vi "第六题a.vi"() -> ()   [LabVIEW 2017]
panel:
  in  "停止 2":bool
  out "显示面板":T1 {"油量" scale=0.0..10.0; "转速（转/秒）" scale=0.0..10000.0; "时速（公里/小时）" scale=0.0..280.0}
  in  "控制面板":T2 {"档位" scale=0.0..10.0; "油门" scale=0.0..100.0}
  out "鞍点":string
  out "随机数数组":dbl[][](array[numeric])
  out "字符串":string
  out "报警灯":bool
  in  "开启报警":bool
  in  "报警上线":dbl(slide) scale=0.0..100.0
  out "温度计":dbl(slide) scale=0.0..100.0
  in  "停止":bool
  # "第二题"
  # "第一题"
  # "第三题"
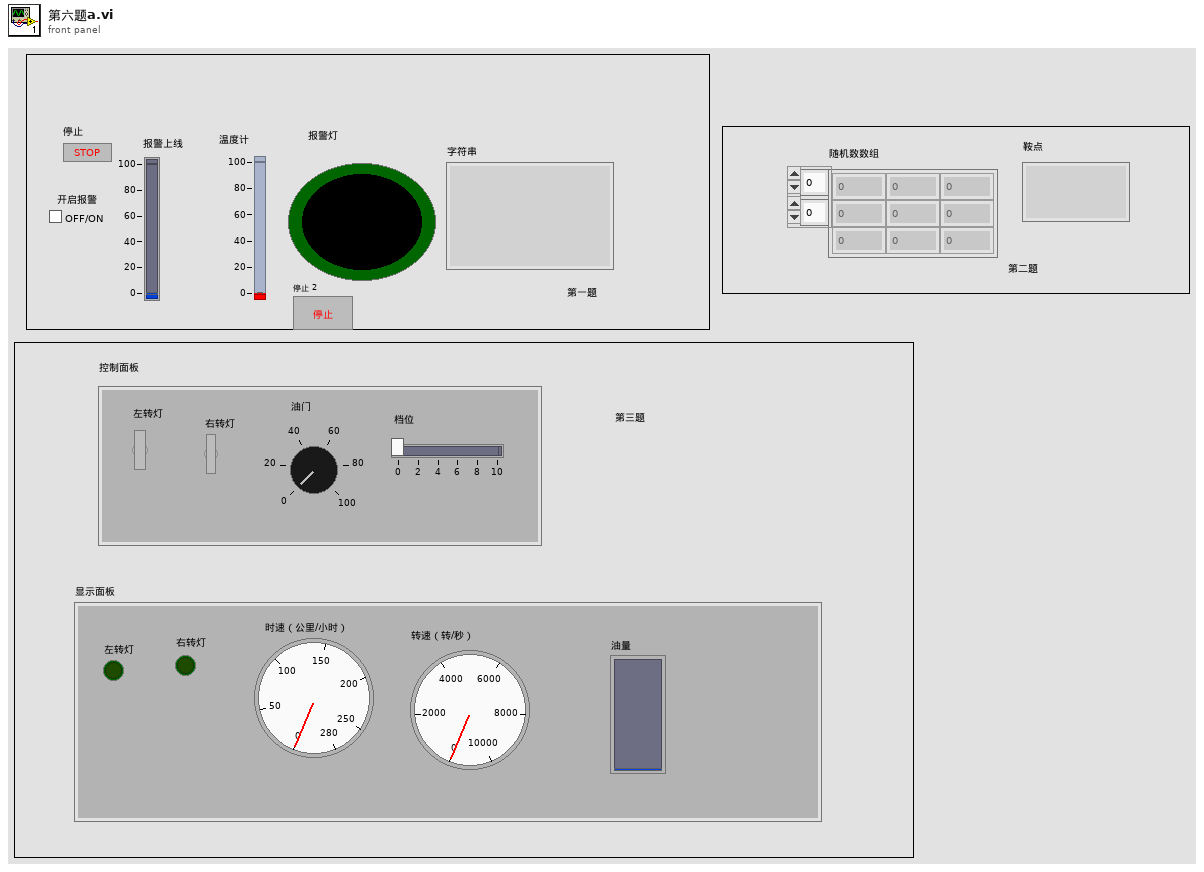
[diagram p1: front panel]
types:
  T1 = cluster{"左转灯":bool, "右转灯":bool, "时速（公里/小时）":dbl, "转速（转/秒） ":dbl, "油量":dbl}
  T2 = cluster{"左转灯":bool, "右转灯":bool, "油门":dbl, "档位":dbl}
  T3 = cluster{"左转灯":bool, "右转灯":bool, dbl, dbl, "b":dbl}
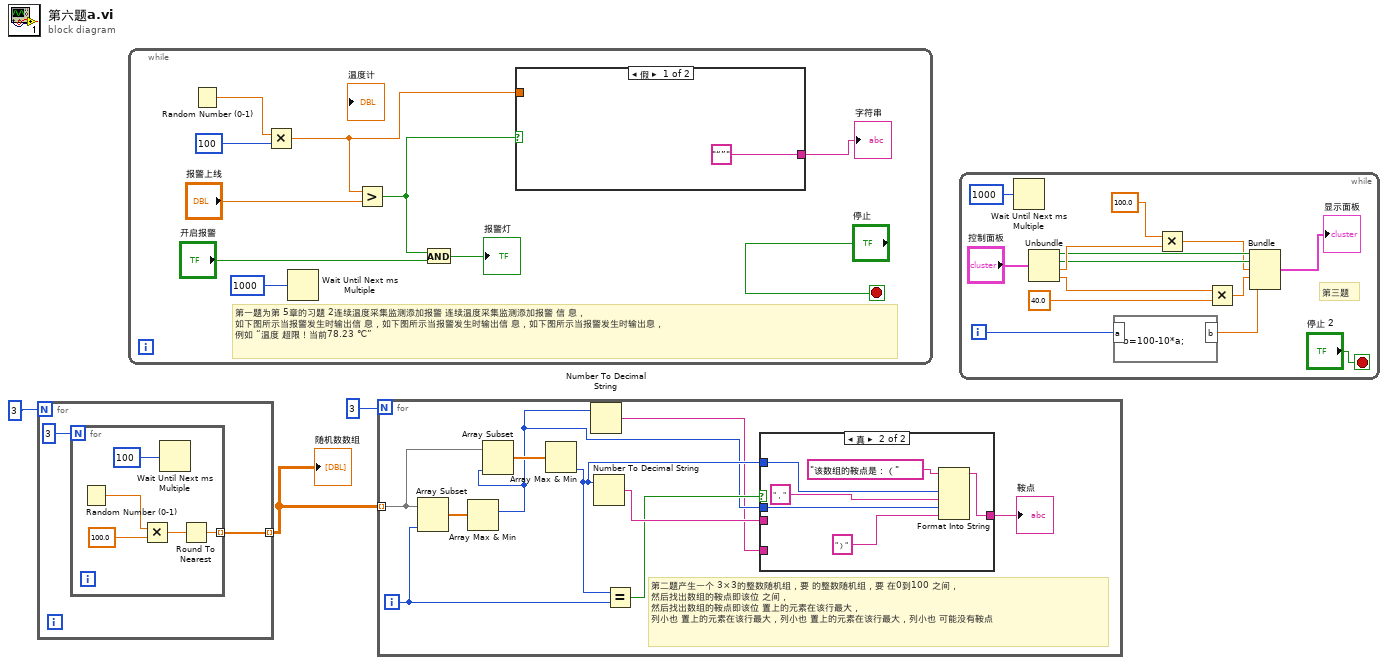
[diagram p0: block diagram]
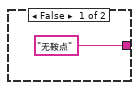
[diagram p2: hidden frame]
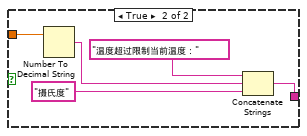
[diagram p3: hidden frame]
diagram:
  n1 = for {
    N: 3 -> [_]
    tunnel: [w4] -> w2 mode=indexing
    n2 = for {
      N: 3 -> [_]
      tunnel: [w6] -> w4 mode=indexing
      n3 = Random Number (0-1)() -> (number: 0 to 1=w9:dbl)
      n4 = Multiply(x=w9, y=100.0) -> (x*y=w7:dbl)
      n5 = Wait Until Next ms Multiple(millisecond multiple=100) -> ()  [unwired: 1 out]
      n6 = Round To Nearest(number=w7) -> (nearest integer value=w6:dbl)
    }
  }
  "随机数数组" <- w2
  n7 = while {
    stop <- "停止" stop-if-true
    # "第一题为第 5章的习题 2连续温度采集监测添加报警 连续温度采集监测添加报警 信 息，\n如下图所示当报警发生时输出信 息，如下图所示当报警发生时输出信 息，如下图所示当报警发生时输出息，\n例如 “温度 超限！当前78.23 ℃”"
    n8 = Random Number (0-1)() -> (number: 0 to 1=w19:dbl)
    n9 = Multiply(x=w19, y=100) -> (x*y=w17:dbl)
    n10 = Wait Until Next ms Multiple(millisecond multiple=1000) -> ()  [unwired: 1 out]
    n11 = Greater?(x=w17, y="报警上线") -> (0:w14:bool)
    n12 = And(x=w14, y="开启报警") -> (x .and. y?=→"报警灯":bool)
    n13 = case shown="假" w14 {
      tunnel: w17 -> [_ w26]
      tunnel: ["“”" w22] -> w11
      frame False {
      }
      frame True {
        n14 = Number To Decimal String(number=w26) -> (decimal integer string=w24:string)  [unwired: 1 in]
        n15 = Concatenate Strings("温度超过限制当前温度：", w24, "摄氏度") -> (w22:string)
      }
    }
    "字符串" <- w11
  }
  n16 = for {
    N: 3 -> [_]
    tunnel: w2 -> [w34] mode=indexing
    i -> [w36]
    # "第二题产生一个 3×3的整数随机组，要 的整数随机组，要 在0到100 之间，\n然后找出数组的鞍点即该位 之间，\n然后找出数组的鞍点即该位 置上的元素在该行最大，\n列小也 置上的元素在该行最大，列小也 置上的元素在该行最大，列小也 可能没有鞍点"
    n17 = Array Subset(array=w34, length=w36) -> (w35:dbl[])  [unwired: 1 in]
    n18 = Array Max & Min(array=w35) -> (max index (indices)=w29:i32)  [unwired: 3 out]
    n19 = Array Subset(array=w34, length=w29) -> (w33:dbl[])  [unwired: 1 in]
    n20 = Array Max & Min(array=w33) -> (min index (indices)=w30:i32)  [unwired: 3 out]
    n21 = Number To Decimal String(number=w29) -> (decimal integer string=w28:string)  [unwired: 1 in]
    n22 = Number To Decimal String(number=w30) -> (decimal integer string=w32:string)  [unwired: 1 in]
    n23 = Equal?(x=w30, y=w36) -> (x = y?=w31:bool)
    n24 = case shown="真" w31 {
      tunnel: w32 -> [_ _]
      tunnel: w30 -> [_ w43]
      tunnel: w29 -> [_ w42]
      tunnel: w28 -> [_ _]
      tunnel: ["无鞍点" w38] -> w27
      frame False {
      }
      frame True {
        n25 = Format Into String(initial string="该数组的鞍点是：（", w43, "，", w42, "）") -> (resulting string=w38:string)  [unwired: 2 in, 1 out]
      }
    }
    "鞍点" <- w27
  }
  n26 = while {
    i -> [w47]
    stop <- "停止 2" stop-if-true
    # "第三题"
    n27 = Wait Until Next ms Multiple(millisecond multiple=1000) -> ()  [unwired: 1 out]
    n28 = Unbundle("控制面板") -> ("左转灯"=w51:bool, "右转灯"=w50:bool, "油门"=w54:dbl, "档位"=w53:dbl)
    n29 = formula code="b=100-10*a;"("a"=w47) -> ("b"=w46:dbl)
    n30 = Multiply(x=100.0, y=w54) -> (x*y=w48:dbl)
    n31 = Multiply(x=w53, y=40.0) -> (x*y=w49:dbl)
    n32 = Bundle("左转灯"=w51, "右转灯"=w50, w48, w49, "b"=w46) -> (→"显示面板":T3)  [unwired: 1 in]
  }
